vi "meas_gui.vi"() -> ()   [LabVIEW 2015]
doc: "Copyright (c) 2018 Frans Korhonen, Institute for Atmospheric and Earth System Research / Physics, Faculty of Science, University of Helsinki, Finland\n\nThis file is part of MeasGUI.\n\nThis Source Code Form is subject to the terms of the Mozilla Public\nLicense, v. 2.0. If a copy of the MPL was not distributed with this\n file, You can obtain one at http://mozilla.org/MPL/2.0/."
uses:
  <vilib>/Math Plots/3D Math Plots/3D Surface/3D Surface XCtrl/3D Surface.xctl
  <vilib>/Platform/TimedLoop/XDataNode/timing_clust.ctl
  <vilib>/Platform/TimedLoop/XDataNode/nitl_modes.ctl
  <vilib>/Platform/TimedLoop/XDataNode/wakeup.ctl
  <vilib>/Math Plots/3D Math Plots/3D Surface/3D Surface Datatype/Public/Plot Helper (Vector).vi
  <vilib>/platform/TimedLoop/XDataNode/XDataNode.xnode
  <vilib>/Math Plots/3D Math Plots/3D Surface/3D Surface Datatype/3D Surface Datatype.lvclass
  <vilib>/Platform/TimedLoop/XDataNode/XDNodeRunTimeDep.lvlib
  draw_to_matlab.vi
panel:
  out "logged controls":refnum<vi>[](array[refnum])
  out "scan start":u32
  out "program path":path
  out "plot channels":string[](array[string])
  out "graph history":T1(array[cluster])
  out "latest graph data":T1(array[cluster])
  out "saved controls":string[](array[string])=["measurement channels", "measurement comments", "measurement parameters", "measurement settings", "measurement logging", "connection settings", "X channel", "Y channels", "Log x", "Log y", "save measurement", "measurement start commands", "measurement end commands"]
  in  "Tab Control":T2(tab)
  in  "open program folder":bool
  in  "file cluster":T3={"Load"=FALSE, "Save"=FALSE, "Configuration"="test"}
  out "set values":string[][](array[string])
  out "latest":string[](array[string])
  in  "run parameters":T4={"save measurement"=TRUE, "stop count"=0}
  out "graph":T1(graph)=[{"measurement data"=[1.0, 2.333333333333333, 3.6666666666666665, 5.0], "measurement data"=[0.0, 0.0, 0.0, 0.0]}]
  out "start time":timestamp=timestamp(3520583178.0378933 s since 1904-01-01) format="%<%H:%M:%S %p %d.%m.%Y>T"
  in  "Measure":bool
  in  "pause":bool
  in  "stop":bool
  in  "scan":T5(array[cluster])=[{"end"=5.0, "start/single"=1.0, "steps"=5, "list"=[], "measurement type"=1, "set channel"="x"}] {"measurement type" items=["Single", "Linear ramp", "Logarithmic ramp", "Chosen list"]; "list" format="%#_6p"; "start/single" format="%#_6p"; "end" format="%#_6p"}
  out "total steps":i32
  in  "plot to Matlab":bool
  in  "scatter to Matlab":bool
  in  "measurement parameters":T6={"startup wait"=0.0, "settling time"=1.0, "total meas time"=10.0, "meas time"=0.0, "dimensons"=1}
  in  "graph parameters":T7={"X channel"=1, "Y channels"=[2], "Log y"=FALSE, "graph history"=0, "Log x"=FALSE, "auto update"=FALSE} {"Y channels" items=["elapsed", "x", "ad1", "r"]; "X channel" items=["elapsed", "x", "ad1", "r"]}
  out "late from schedule":dbl
  in  "record channels":string[](array[string])
  in  "measurement comments":string="these are the comments for the measurement\nsecond line"
  in  "measurement start commands":string
  in  "measurement end commands":string
  in  "measurement logging":T8={"measurement file"="data\\meas_%Y%m%d", "column separator"=";"}
  in  "next configuration":T9={"load next"=FALSE, "next configuration"="test"}
  out "data":string
  in  "Configure measurement devices":bool
  in  "Configure local hardware":bool
  in  "connection settings":T10={"Serial port"="COM1", "Network address"="192.168.10.15", "connection method"=enum."SERIAL (VISA)", "Port"=1300, "Pipe name"="\\\\.\\pipe\\channel_system"}
  in  "3D graph parameters":T11={"3D X channel"=1, "3D Y channel"=2, "3D Z channel"=3, "auto update"=FALSE} {"3D Z channel" items=["elapsed", "x", "ad1", "r"]; "3D Y channel" items=["elapsed", "x", "ad1", "r"]; "3D X channel" items=["elapsed", "x", "ad1", "r"]}
  out "3D Surface":refnum<class "3D Plot Datatype.lvclass">[](xcontrol)
  in  "draw to matlab":bool
  out "measurement data":dbl[][](array[numeric]) format="%#_3p"
  out "measurement channels":string[](array[string])
  # "click on graph to update manually"
  # "time indicators in filename:\n%Y = year\n%m = month\n%d = day\n%H = hour\n%M = minute\n%S = second"
  # "ms"
  # "0 = dont stop"
  # "+(.csv & .log)"
  # "click on graph to update"
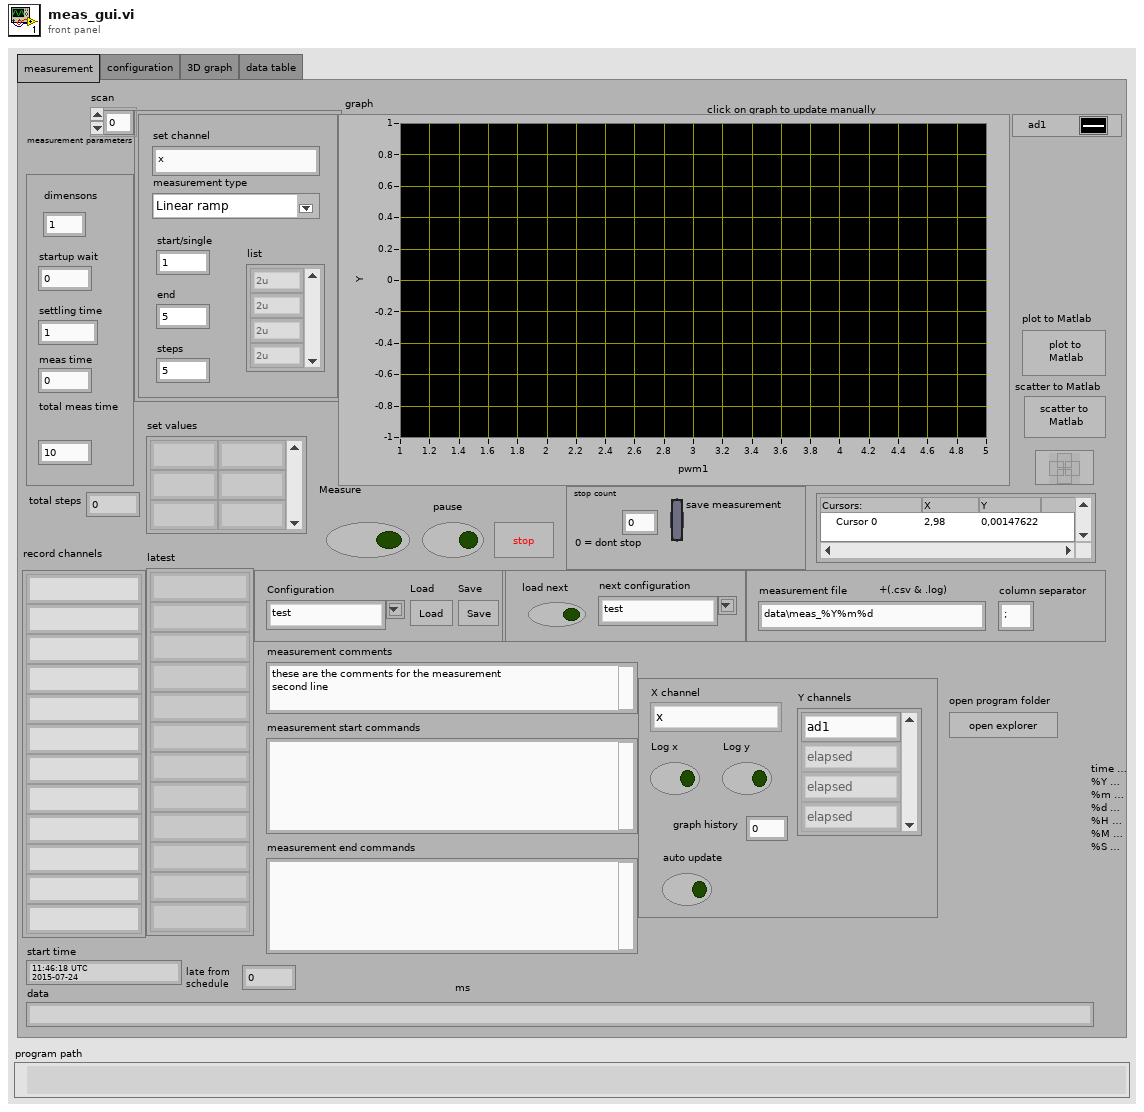
[diagram p1: front panel]
types:
  T1 = cluster{"measurement data":dbl[], "measurement data":dbl[]}[]
  T2 = enum32{"measurement", "configuration", "3D graph", "data table"}
  T3 = cluster{"Load":bool, "Save":bool, "Configuration":string}
  T4 = cluster{"save measurement":bool, "stop count":u32}
  T5 = cluster{"end":dbl, "start/single":dbl, "steps":i32, "list":dbl[], "measurement type":u16, "set channel":string}[]
  T6 = cluster{"startup wait":dbl, "settling time":dbl, "total meas time":dbl, "meas time":dbl, "dimensons":i32}
  T7 = cluster{"X channel":u16, "Y channels":u16[], "Log y":bool, "graph history":i32, "Log x":bool, "auto update":bool}
  T8 = cluster{"measurement file":string, "column separator":string}
  T9 = cluster{"load next":bool, "next configuration":string}
  T10 = cluster{"Serial port":refnum<visa-resource-name>, "Network address":string, "connection method":enum16{"SERIAL (VISA)", "UDP", "LOCAL", "PIPE", "SERIAL (pipe channel)"}, "Port":u16, "Pipe name":string}
  T11 = cluster{"3D X channel":u16, "3D Y channel":u16, "3D Z channel":u16, "auto update":bool}
  T12 = enum16{"open", "replace", "create", "open or create", "replace or create", "replace or create with confirmation"}
  T13 = enum16{"SERIAL (VISA)", "UDP", "LOCAL", "PIPE", "SERIAL (pipe channel)"}
  T14 = cluster{"measurement data":dbl[], "measurement data":dbl[]}
  T15 = enum16{"read", "write", "reset", "conf", "link", "raw communication"}
  T16 = typedef "XDNodeRunTimeDep.lvlib/timing_clust.ctl" = cluster{"Expected End [f-1]":u64, "Actual End [f-1]":u64, "Finished Late? [f-1]":bool, "Expected End [i-1]":u64, "Actual End [i-1]":u64, "Finished Late? [i-1]":bool, "Expected Start [i]":u64, "Actual Start [i]":u64, "Expected Start [f]":u64, "Actual Start [f]":u64, "Source Name":string, "Structure Name":string, "Period":i64, "Deadline":i64, "Offset":i64, "Start":i64, "Priority":i32, "Timeout":i32, "Mode":T17, "Wakeup Reason":T18, "Error":errorcluster, "Source Type":string, "Secondary Source Type":string, "Global End Time":u64, "Global Start Time":u64, "Frame Duration":u64, "Iteration Duration":u64, "Assigned CPU":i32, "I/O Scan Engine Mode":u32}
  T17 = typedef "XDNodeRunTimeDep.lvlib/nitl_modes.ctl" = enum32{"No Change", "Process missed periods, maintain original phase", "Discard missed periods, maintain original phase", "Process missed periods, ignore original phase", "Discard missed periods, ignore original phase"}
  T18 = typedef "XDNodeRunTimeDep.lvlib/wakeup.ctl" = enum32{"Normal", "Aborted", "Asynchronous wakeup", "Timing source error", "Timed loop error", "Timeout"}
  T19 = cluster{"end":dbl, "start/single":dbl, "steps":i32, "list":dbl[], "measurement type":u16, "set channel":string}
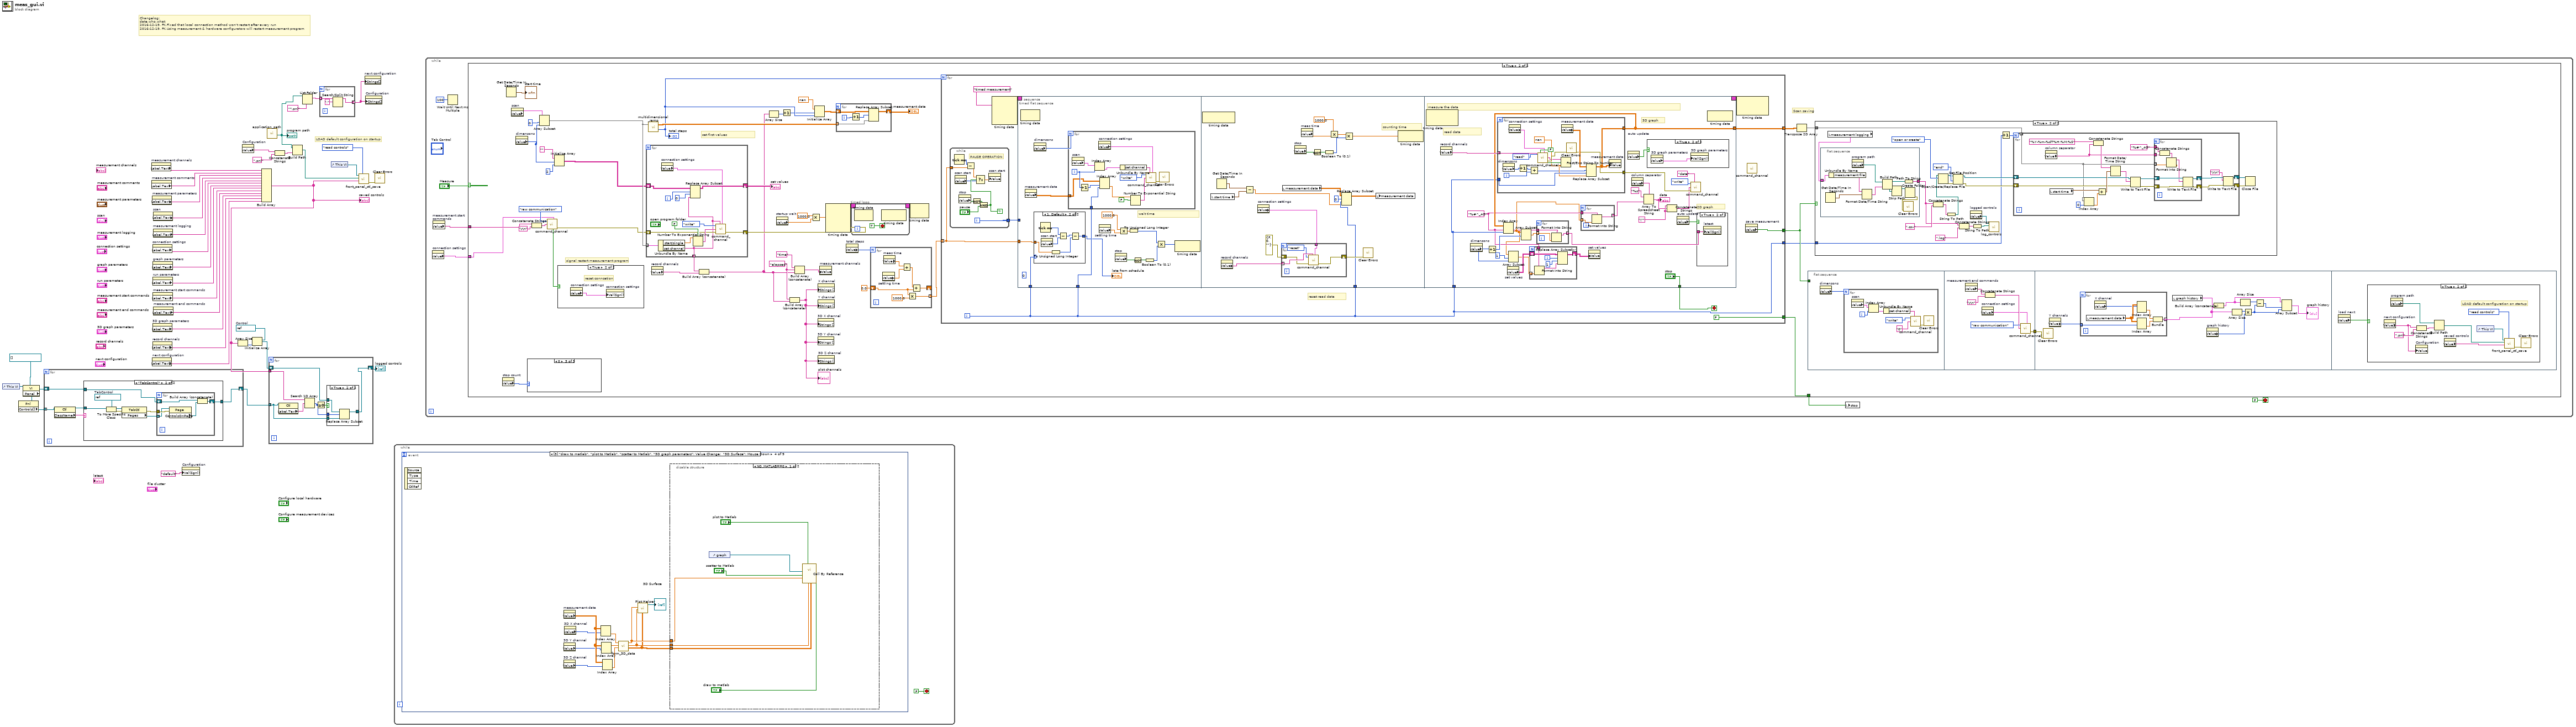
[diagram p0: block diagram]
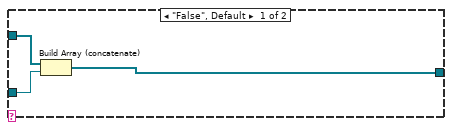
[diagram p3: hidden frame]
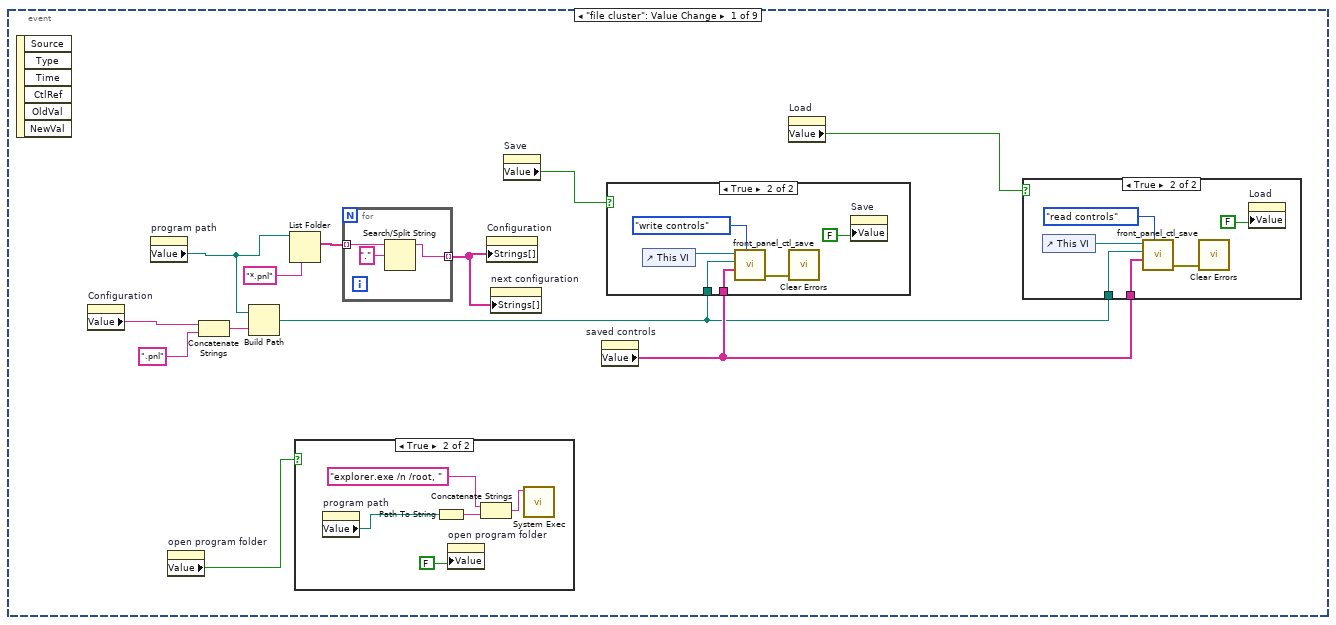
[diagram p4: hidden frame]
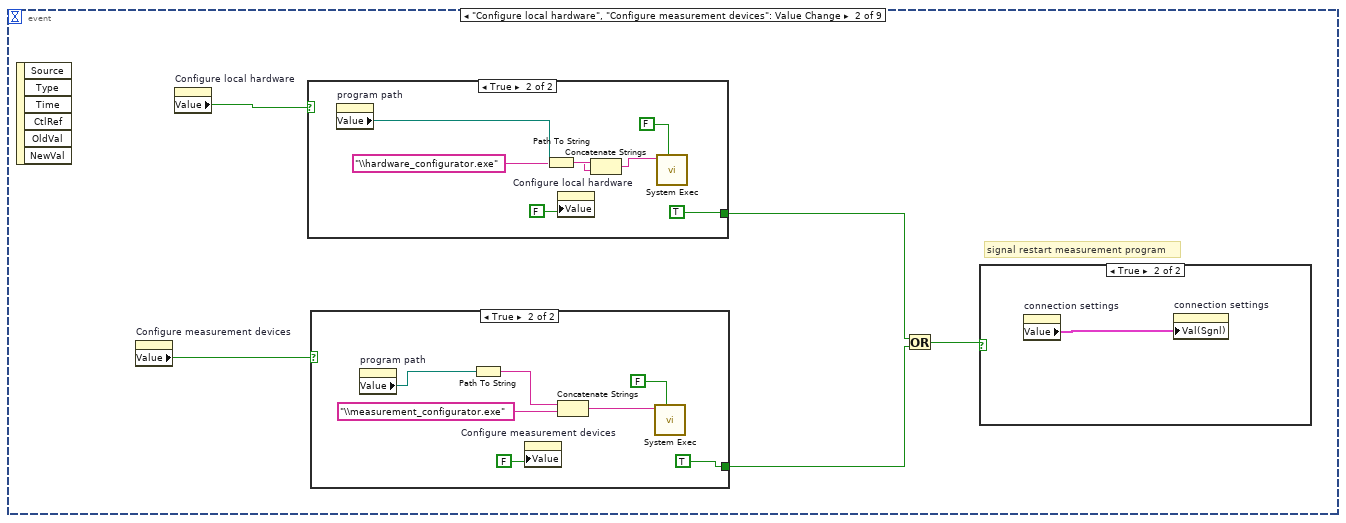
[diagram p8: hidden frame]
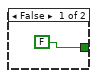
[diagram p10: hidden frame]
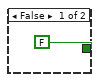
[diagram p11: hidden frame]
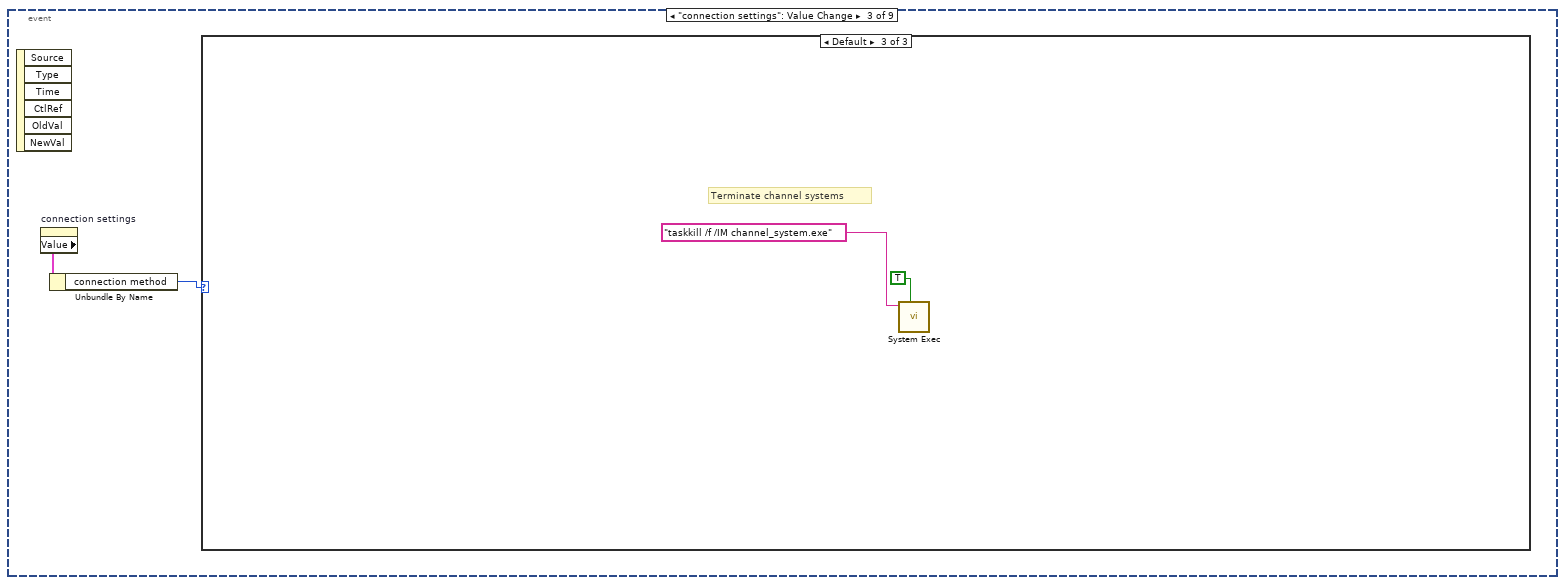
[diagram p12: hidden frame]
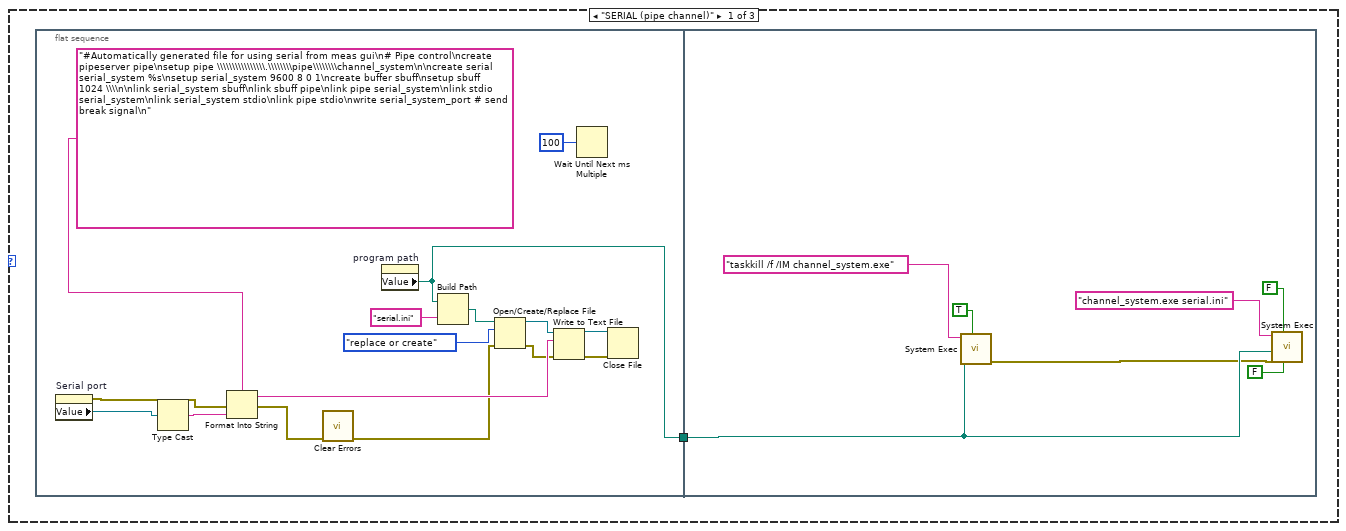
[diagram p13: hidden frame]
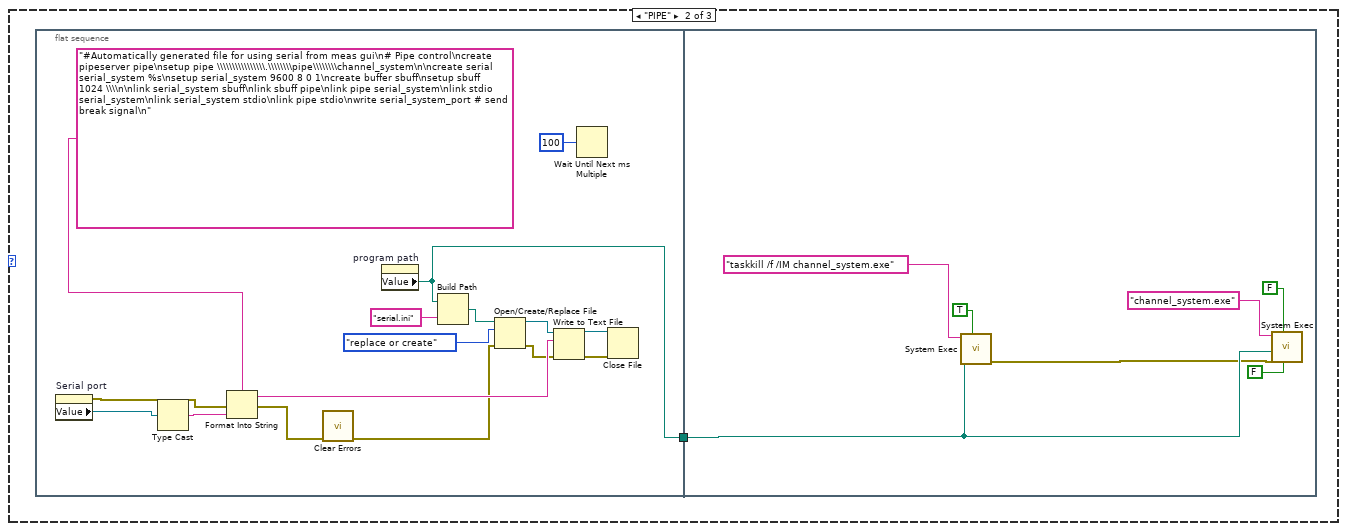
[diagram p14: hidden frame]
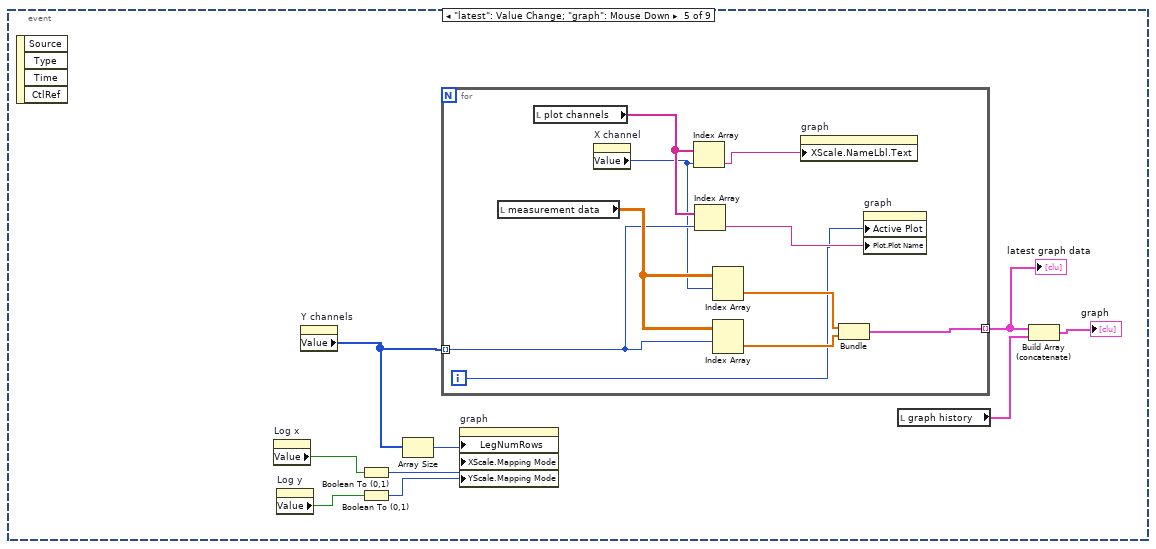
[diagram p16: hidden frame]
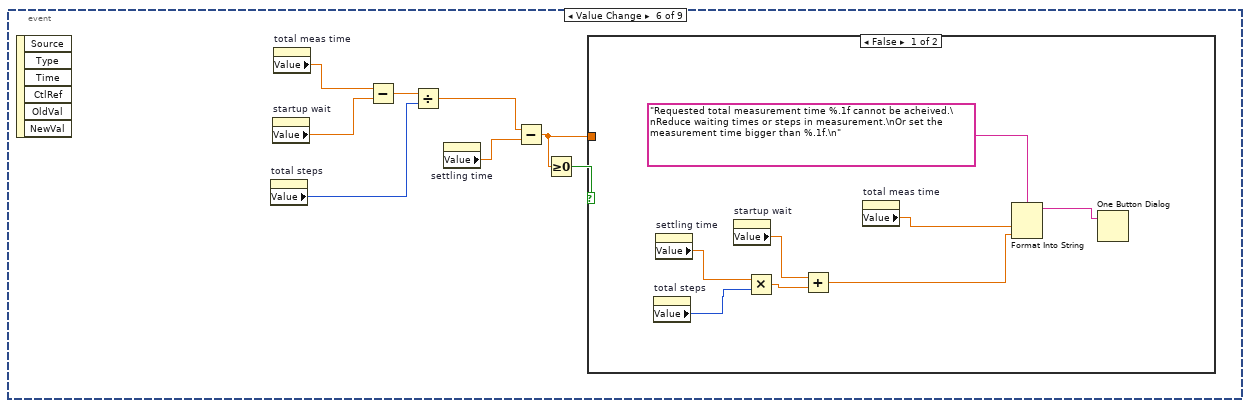
[diagram p17: hidden frame]
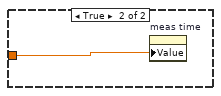
[diagram p18: hidden frame]
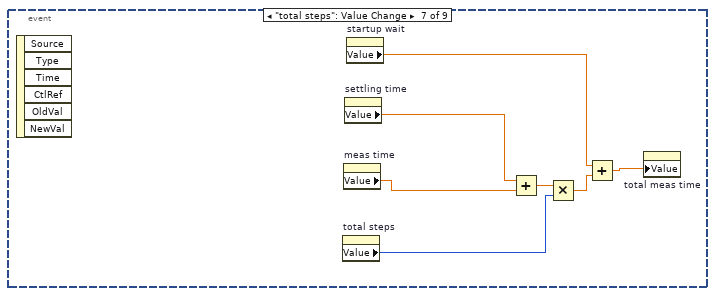
[diagram p19: hidden frame]
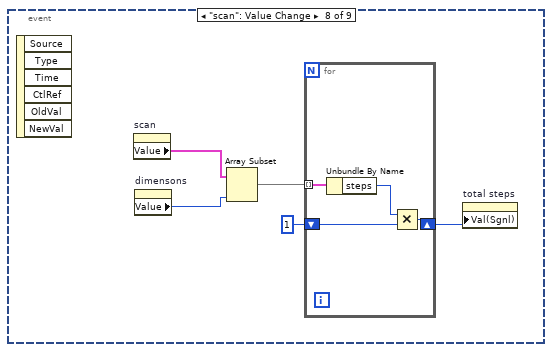
[diagram p20: hidden frame]
diagram:
  w10 = refnum<vi> refnum  # Control
  # "Changelog: \ndate,who,what\n2016-12-19. FK,Fixed that local connection method won't restart after every run\n2016-12-19. FK,Using measurement & hardware configurators will restart measurement program"
  # "LOAD default configuration on startup"
  n1 = control-ref of="This VI"() -> (w17:refnum<vi>)
  n2 = property on="Property Node" class="VI"(reference=w17) -> ("Panel"=w16:refnum<vi>)  [unwired: 1 in, 2 out]
  n3 = property class="Pnl"(reference=w16) -> ("Controls[]"=w15:refnum<vi>[])  [unwired: 1 in, 2 out]
  n4 = for {
    tunnel: w15 -> [w40] mode=indexing
    shift-right: [w37] -> w13
    shift-left: refnum<vi>[] [] -> [w36]
    n5 = property class="Ctl"(reference=w40) -> (reference out=w38:refnum<vi>, "ClassName"=w39:string)  [unwired: 1 in, 1 out]
    n6 = case shown="\"TabControl\"" w39 {
      tunnel: w38 -> [w42 w51]
      tunnel: [w41 w45] -> w37
      tunnel: w36 -> [w43 w44]
      frame "False", Default {
        n7 = Build Array (concatenate)(w43, w42) -> (w41:refnum<vi>[])
      }
      frame "TabControl" {
        w50 = refnum<vi> refnum  # TabControl
        n8 = To More Specific Class(target class=w50, reference=w51) -> (specific class reference=w49:refnum<vi>, error out=w48:errorcluster)  [unwired: 1 in]
        n9 = property class="TabCtl"(reference=w49, error in=w48) -> (error out=w47:errorcluster, "Pages"=w46:refnum<vi>[])  [unwired: 1 out]
        n10 = for {
          tunnel: w47 -> [w56]
          tunnel: w46 -> [w55] mode=indexing
          shift-right: [w53] -> w45
          shift-left: w44 -> [w52]
          n11 = property class="Page"(reference=w55, error in=w56) -> ("ControlsOnPage"=w54:refnum<vi>[])  [unwired: 2 out]
          n12 = Build Array (concatenate)(w52, w54) -> (w53:refnum<vi>[])
        }
      }
    }
  }
  n13 = property on="measurement channels" class="Arr (strict)"() -> ("Label.Text"=w29:string)  [unwired: 2 in, 2 out]
  n14 = property on="measurement comments" class="Str"() -> ("Label.Text"=w27:string)  [unwired: 2 in, 2 out]
  n15 = property on="measurement parameters" class="Clust (strict)"() -> ("Label.Text"=w26:string)  [unwired: 2 in, 2 out]
  n16 = property on="next configuration" class="Clust (strict)"() -> ("Label.Text"=w2:string)  [unwired: 2 in, 2 out]
  n17 = property on="connection settings" class="Clust (strict)"() -> ("Label.Text"=w3:string)  [unwired: 2 in, 2 out]
  n18 = property on="3D graph parameters" class="Clust (strict)"() -> ("Label.Text"=w19:string)  [unwired: 2 in, 2 out]
  n19 = property on="record channels" class="Arr (strict)"() -> ("Label.Text"=w18:string)  [unwired: 2 in, 2 out]
  n20 = property on="graph parameters" class="Clust (strict)"() -> ("Label.Text"=w23:string)  [unwired: 2 in, 2 out]
  n21 = property on="run parameters" class="Clust (strict)"() -> ("Label.Text"=w22:string)  [unwired: 2 in, 2 out]
  n22 = property on="measurement start commands" class="Str"() -> ("Label.Text"=w21:string)  [unwired: 2 in, 2 out]
  n23 = property on="scan" class="Arr (strict)"() -> ("Label.Text"=w25:string)  [unwired: 2 in, 2 out]
  n24 = property on="measurement logging" class="Clust (strict)"() -> ("Label.Text"=w24:string)  [unwired: 2 in, 2 out]
  n25 = property on="measurement end commands" class="Str"() -> ("Label.Text"=w20:string)  [unwired: 2 in, 2 out]
  n26 = property on="Configuration" class="CmbBox"("Val(Sgnl)"="default" ("Value (Signaling)")) -> ()  [unwired: 2 in, 2 out]
  n27 = property on="Configuration" class="CmbBox"() -> ("Value"=w28:string)  [unwired: 2 in, 2 out]
  n28 = Build Array(w29, w27, w26, w25, w24, w3, w23, w22, w21, w20, w19, w18, w2) -> (w12:string[])
  "saved controls" <- w12
  n29 = Array Size(array=w12) -> (size(s)=w11:i32)
  n30 = Initialize Array(w10, w11) -> (w9:refnum<vi>[])
  n31 = call "application_path.vi"() -> ("path"=w4:path)  [unwired: 11 in]
  "program path" <- w4
  n32 = for {
    tunnel: w13 -> [w59] mode=indexing
    tunnel: w12 -> [w62]
    shift-right: [w58] -> w8
    shift-left: w9 -> [w57]
    n33 = property class="Ctl"(reference=w59) -> ("Label.Text"=w63:string)  [unwired: 1 in, 2 out]
    n34 = Search 1D Array(1D array=w62, element=w63) -> (index of element=w60:i32)  [unwired: 1 in]
    n35 = Greater Or Equal To 0?(x=w60) -> (x >= 0?=w61:bool)
    n36 = case shown="True" w61 {
      tunnel: w60 -> [_ w68]
      tunnel: w59 -> [_ w67]
      tunnel: [w64 w66] -> w58
      tunnel: w57 -> [w64 w65]
      frame False {
      }
      frame True {
        n37 = Replace Array Subset(array=w65, new element=w67, index=w68) -> (w66:refnum<vi>[])
      }
    }
  }
  "logged controls" <- w8
  n38 = Concatenate Strings(w28, ".pnl" ("string")) -> (w34:string)
  n39 = Build Path(base path=w4, name or relative path=w34) -> (appended path=w31:path)
  n40 = List Folder(path=w4, pattern="*.pnl") -> (filenames=w5:string[])  [unwired: 2 in, 3 out]
  n41 = for {
    tunnel: w5 -> [w71] mode=indexing
    tunnel: [w70] -> w1 mode=indexing
    n42 = Search/Split String(string=w71, search string/char (-)=".") -> (substring before match=w70:string)  [unwired: 1 in, 2 out]
  }
  n43 = control-ref of="This VI"() -> (w30:refnum<vi>)
  n44 = call "front_panel_ctl_save.vi"("VI in"=w30, "method"=enum16{"read controls", "write controls"}."read controls", "filename"=w31, "controls"=w12) -> ("error out"=w33:errorcluster)  [unwired: 4 in]
  n45 = property on="next configuration" class="CmbBox"("Strings[]"=w1) -> ()  [unwired: 2 in, 2 out]
  n46 = property on="Configuration" class="CmbBox"("Strings[]"=w1) -> ()  [unwired: 2 in, 2 out]
  n47 = call <vilib>:"Clear Errors.vi"("error in (no error)"=w33) -> ()  [unwired: 5 in, 2 out]
  n48 = while {
    stop <- FALSE stop-if-true
    n49 = event shown="[3] \"draw to matlab\", \"plot to Matlab\", \"scatter to Matlab\", \"3D graph parameters\": Value Change;  \"3D Surface\": Mouse Down" {
      selector: _ -> [_ _ _ _ _ _ _ _ _]
      dyn-events: _ -> [_ _ _ _ _ _ _ _ _]
      timeout: _ -> [_ _ _ _ _ _ _ _ _]
      event "file cluster": Value Change {
        n50 = event-data() -> ()  [unwired: 1 in, 6 out]
        n51 = property on="Configuration" class="CmbBox"() -> ("Value"=w77:string)  [unwired: 2 in, 2 out]
        n52 = property on="program path" class="Path"() -> ("Value"=w78:path)  [unwired: 2 in, 2 out]
        n53 = property on="open program folder" class="Bool (strict)"() -> ("Value"=w74:bool)  [unwired: 2 in, 2 out]
        n54 = Concatenate Strings(w77, ".pnl" ("string")) -> (w82:string)
        n55 = Build Path(base path=w78, name or relative path=w82) -> (appended path=w79:path)
        n56 = List Folder(path=w78, pattern="*.pnl") -> (filenames=w81:string[])  [unwired: 2 in, 3 out]
        n57 = case shown="True" w74 {
          frame False {
          }
          frame True {
            n58 = property on="program path" class="Path"() -> ("Value"=w86:path)  [unwired: 2 in, 2 out]
            n59 = Path To String(path=w86) -> (string=w87:string)
            n60 = property on="open program folder" class="Bool (strict)"("Value"=FALSE) -> ()  [unwired: 2 in, 2 out]
            n61 = Concatenate Strings("explorer.exe /n /root, " ("string"), w87) -> (w88:string)
            n62 = call <vilib>:"System Exec.vi"("command line"=w88) -> ()  [unwired: 7 in, 4 out]
          }
        }
        n63 = for {
          tunnel: w81 -> [w92] mode=indexing
          tunnel: [w91] -> w73 mode=indexing
          n64 = Search/Split String(string=w92, search string/char (-)=".") -> (substring before match=w91:string)  [unwired: 1 in, 2 out]
        }
        n65 = property on="Configuration" class="CmbBox"("Strings[]"=w73) -> ()  [unwired: 2 in, 2 out]
        n66 = property on="next configuration" class="CmbBox"("Strings[]"=w73) -> ()  [unwired: 2 in, 2 out]
        n67 = property on="Save" class="Bool (strict)"() -> ("Value"=w75:bool)  [unwired: 2 in, 2 out]
        n68 = property on="saved controls" class="Arr (strict)"() -> ("Value"=w80:string[])  [unwired: 2 in, 2 out]
        n69 = case shown="True" w75 {
          tunnel: w80 -> [_ w102]
          tunnel: w79 -> [_ w101]
          frame False {
          }
          frame True {
            n70 = control-ref of="This VI"() -> (w104:refnum<vi>)
            n71 = call "front_panel_ctl_save.vi"("VI in"=w104, "method"=enum16{"read controls", "write controls"}."write controls", "filename"=w101, "controls"=w102) -> ("error out"=w99:errorcluster)  [unwired: 4 in]
            n72 = call <vilib>:"Clear Errors.vi"("error in (no error)"=w99) -> ()  [unwired: 5 in, 2 out]
            n73 = property on="Save" class="Bool (strict)"("Value"=FALSE) -> ()  [unwired: 2 in, 2 out]
          }
        }
        n74 = property on="Load" class="Bool (strict)"() -> ("Value"=w76:bool)  [unwired: 2 in, 2 out]
        n75 = case shown="True" w76 {
          tunnel: w80 -> [_ w95]
          tunnel: w79 -> [_ w96]
          frame False {
          }
          frame True {
            n76 = control-ref of="This VI"() -> (w97:refnum<vi>)
            n77 = call "front_panel_ctl_save.vi"("VI in"=w97, "method"=enum16{"read controls", "write controls"}."read controls", "filename"=w96, "controls"=w95) -> ("error out"=w93:errorcluster)  [unwired: 4 in]
            n78 = call <vilib>:"Clear Errors.vi"("error in (no error)"=w93) -> ()  [unwired: 5 in, 2 out]
            n79 = property on="Load" class="Bool (strict)"("Value"=FALSE) -> ()  [unwired: 2 in, 2 out]
          }
        }
      }
      event "Configure local hardware", "Configure measurement devices": Value Change {
        # "signal restart measurement program"
        n80 = event-data() -> ()  [unwired: 1 in, 6 out]
        n81 = property on="Configure measurement devices" class="Bool (strict)"() -> ("Value"=w108:bool)  [unwired: 2 in, 2 out]
        n82 = property on="Configure local hardware" class="Bool (strict)"() -> ("Value"=w109:bool)  [unwired: 2 in, 2 out]
        n83 = case shown="True" w109 {
          tunnel: [FALSE TRUE] -> w106
          frame False {
          }
          frame True {
            n84 = property on="program path" class="Path"() -> ("Value"=w124:path)  [unwired: 2 in, 2 out]
            n85 = Path To String(path=w124) -> (string=w125:string)
            n86 = property on="Configure local hardware" class="Bool (strict)"("Value"=FALSE) -> ()  [unwired: 2 in, 2 out]
            n87 = Concatenate Strings(w125, "\\hardware_configurator.exe" ("string")) -> (w126:string)
            n88 = call <vilib>:"System Exec.vi"("wait until completion? (T)"=FALSE, "command line"=w126) -> ()  [unwired: 6 in, 4 out]
          }
        }
        n89 = case shown="True" w108 {
          tunnel: [FALSE TRUE] -> w105
          frame False {
          }
          frame True {
            n90 = property on="program path" class="Path"() -> ("Value"=w115:path)  [unwired: 2 in, 2 out]
            n91 = Path To String(path=w115) -> (string=w114:string)
            n92 = property on="Configure measurement devices" class="Bool (strict)"("Value"=FALSE) -> ()  [unwired: 2 in, 2 out]
            n93 = Concatenate Strings(w114, "\\measurement_configurator.exe" ("string")) -> (w118:string)
            n94 = call <vilib>:"System Exec.vi"("wait until completion? (T)"=FALSE, "command line"=w118) -> ()  [unwired: 6 in, 4 out]
          }
        }
        n95 = Or(x=w106, y=w105) -> (x .or. y?=w107:bool)
        n96 = case shown="True" w107 {
          frame False {
          }
          frame True {
            n97 = property on="connection settings" class="Clust (strict)"() -> ("Value"=w110:T10)  [unwired: 2 in, 2 out]
            n98 = property on="connection settings" class="Clust (strict)"("Val(Sgnl)"=w110) -> ()  [unwired: 2 in, 2 out]
          }
        }
      }
      event "connection settings": Value Change {
        n99 = event-data() -> ()  [unwired: 1 in, 6 out]
        n100 = property on="connection settings" class="Clust (strict)"() -> ("Value"=w128:T10)  [unwired: 2 in, 2 out]
        n101 = Unbundle By Name(w128) -> ("connection method"=w127:T13)
        n102 = case shown="Default" w127 {
          frame "SERIAL (pipe channel)" {
            n103 = flat-sequence {
              tunnel: [w131] -> w129
              tunnel: w129 -> [w147]
              frame #0 {
                n104 = property on="Serial port" class="VISAName"() -> (error out=w138:errorcluster, "Value"=w136:refnum<visa-resource-name>)  [unwired: 2 in, 1 out]
                n105 = Type Cast(x=w136) -> (*(type *) &x=w137:string)  [unwired: 1 in]
                n106 = Format Into String(format string="#Automatically generated file for using serial from meas gui\n# Pipe control\ncreate pipeserver pipe\nsetup pipe \\\\\\\\\\\\\\\\.\\\\\\\\pipe\\\\\\\\channel_system\n\ncreate serial serial_system %s\nsetup serial_system 9600 8 0 1\ncreate buffer sbuff\nsetup sbuff 1024 \\\\n\nlink serial_system sbuff\nlink sbuff pipe\nlink pipe serial_system\nlink stdio serial_system\nlink serial_system stdio\nlink pipe stdio\nwrite serial_system_port # send break signal\n", error in=w138, w137) -> (resulting string=w144:string, error out=w139:errorcluster)  [unwired: 1 in]
                n107 = call <vilib>:"Clear Errors.vi"("error in (no error)"=w139) -> ("error out"=w133:errorcluster)  [unwired: 5 in, 1 out]
                n108 = property on="program path" class="Path"() -> ("Value"=w131:path)  [unwired: 2 in, 2 out]
                n109 = Build Path(base path=w131, name or relative path="serial.ini") -> (appended path=w141:path)
                n110 = Open/Create/Replace File(file path (use dialog)=w141, error in=w133, operation (0:open)=T12."replace or create") -> (refnum out=w143:refnum<file>, error out=w134:errorcluster)  [unwired: 3 in, 1 out]
                n111 = Write to Text File(file (use dialog)=w143, text=w144, error in=w134) -> (refnum out=w145:refnum<file>, error out=w135:errorcluster)  [unwired: 1 in, 1 out]
                n112 = Wait Until Next ms Multiple(millisecond multiple=u32 100) -> ()  [unwired: 1 out]
                n113 = Close File(refnum=w145, error in=w135) -> ()  [unwired: 2 out]
              }
              frame #1 {
                n114 = call <vilib>:"System Exec.vi"("wait until completion? (T)"=TRUE, "working directory"=w147, "command line"="taskkill /f /IM channel_system.exe") -> ("error out"=w146:errorcluster)  [unwired: 5 in, 3 out]
                n115 = call <vilib>:"System Exec.vi"("run minimized? (F)"=FALSE, "wait until completion? (T)"=FALSE, "error in (no error)"=w146, "working directory"=w147, "command line"="channel_system.exe serial.ini") -> ()  [unwired: 3 in, 4 out]
              }
            }
          }
          frame "PIPE" {
            n116 = flat-sequence {
              tunnel: [w155] -> w153
              tunnel: w153 -> [w171]
              frame #0 {
                n117 = property on="Serial port" class="VISAName"() -> (error out=w162:errorcluster, "Value"=w160:refnum<visa-resource-name>)  [unwired: 2 in, 1 out]
                n118 = Type Cast(x=w160) -> (*(type *) &x=w161:string)  [unwired: 1 in]
                n119 = Format Into String(format string="#Automatically generated file for using serial from meas gui\n# Pipe control\ncreate pipeserver pipe\nsetup pipe \\\\\\\\\\\\\\\\.\\\\\\\\pipe\\\\\\\\channel_system\n\ncreate serial serial_system %s\nsetup serial_system 9600 8 0 1\ncreate buffer sbuff\nsetup sbuff 1024 \\\\n\nlink serial_system sbuff\nlink sbuff pipe\nlink pipe serial_system\nlink stdio serial_system\nlink serial_system stdio\nlink pipe stdio\nwrite serial_system_port # send break signal\n", error in=w162, w161) -> (resulting string=w168:string, error out=w163:errorcluster)  [unwired: 1 in]
                n120 = call <vilib>:"Clear Errors.vi"("error in (no error)"=w163) -> ("error out"=w157:errorcluster)  [unwired: 5 in, 1 out]
                n121 = property on="program path" class="Path"() -> ("Value"=w155:path)  [unwired: 2 in, 2 out]
                n122 = Build Path(base path=w155, name or relative path="serial.ini") -> (appended path=w165:path)
                n123 = Open/Create/Replace File(file path (use dialog)=w165, error in=w157, operation (0:open)=T12."replace or create") -> (refnum out=w167:refnum<file>, error out=w158:errorcluster)  [unwired: 3 in, 1 out]
                n124 = Write to Text File(file (use dialog)=w167, text=w168, error in=w158) -> (refnum out=w169:refnum<file>, error out=w159:errorcluster)  [unwired: 1 in, 1 out]
                n125 = Wait Until Next ms Multiple(millisecond multiple=u32 100) -> ()  [unwired: 1 out]
                n126 = Close File(refnum=w169, error in=w159) -> ()  [unwired: 2 out]
              }
              frame #1 {
                n127 = call <vilib>:"System Exec.vi"("wait until completion? (T)"=TRUE, "working directory"=w171, "command line"="taskkill /f /IM channel_system.exe") -> ("error out"=w170:errorcluster)  [unwired: 5 in, 3 out]
                n128 = call <vilib>:"System Exec.vi"("run minimized? (F)"=FALSE, "wait until completion? (T)"=FALSE, "error in (no error)"=w170, "working directory"=w171, "command line"="channel_system.exe") -> ()  [unwired: 3 in, 4 out]
              }
            }
          }
          frame Default {
            # "Terminate channel systems"
            n129 = call <vilib>:"System Exec.vi"("wait until completion? (T)"=TRUE, "command line"="taskkill /f /IM channel_system.exe") -> ()  [unwired: 6 in, 4 out]
          }
        }
      }
      event "draw to matlab", "plot to Matlab", "scatter to Matlab", "3D graph parameters": Value Change; "3D Surface": Mouse Down {
        n130 = event-data() -> ()  [unwired: 1 in, 4 out]
        n131 = property on="measurement data" class="Arr (strict)"() -> ("Value"=w189:dbl[][])  [unwired: 2 in, 2 out]
        n132 = property on="3D Y channel" class="Ring (strict)"() -> ("Value"=w188:u16)  [unwired: 2 in, 2 out]
        n133 = property on="3D Z channel" class="Ring (strict)"() -> ("Value"=w187:u16)  [unwired: 2 in, 2 out]
        n134 = property on="3D X channel" class="Ring (strict)"() -> ("Value"=w186:u16)  [unwired: 2 in, 2 out]
        n135 = Index Array(array=w189, index (row)=w186) -> (element=w183:dbl[])  [unwired: 1 in]
        n136 = Index Array(array=w189, index (row)=w188) -> (element=w184:dbl[])  [unwired: 1 in]
        n137 = Index Array(array=w189, index (row)=w187) -> (element=w185:dbl[])  [unwired: 1 in]
        n138 = call "form_3D_data.vi"("z data"=w185, "y data"=w184, "x data"=w183) -> ("Z matrix"=w179:dbl[][], "y vector"=w180:dbl[], "x vector"=w181:dbl[])  [unwired: 6 in]
        n139 = call-poly <vilib>:"Plot Helper.vi"("z matrix"=w179, "y vector"=w180, "x vector"=w181) -> ("3D Plot lvclass Array out"=→"3D Surface":refnum<class "3D Plot Datatype.lvclass">[])  [unwired: 3 in, 5 out]
        n140 = disable-structure shown="NO_MATLAB==0" {
          disable-tunnel: w181 -> [w193 _]
          disable-tunnel: w180 -> [w192 _]
          disable-tunnel: w179 -> [w191 _]
          frame condition #0 (active) {
            n141 = control-ref of="graph"() -> (w190:refnum<vi>)
            n142 = call-by-ref "?"("Z matrix"=w191, "draw to matlab"="draw to matlab", "y vector"=w192, "plot to Matlab"="plot to Matlab", "x vector"=w193, "scatter to Matlab"="scatter to Matlab", "XYGraph in"=w190) -> ()  [unwired: 7 in, 2 out]
          }
          frame condition #1 {
          }
        }
      }
      event "latest": Value Change; "graph": Mouse Down {
        n143 = event-data() -> ()  [unwired: 1 in, 4 out]
        n144 = property on="Log x" class="Bool (strict)"() -> ("Value"=w200:bool)  [unwired: 2 in, 2 out]
        n145 = property on="Log y" class="Bool (strict)"() -> ("Value"=w199:bool)  [unwired: 2 in, 2 out]
        n146 = property on="Y channels" class="Arr (strict)"() -> ("Value"=w198:u16[])  [unwired: 2 in, 2 out]
        n147 = Boolean To (0,1)(Boolean=w200) -> (0, 1=w205:i16)
        n148 = Boolean To (0,1)(Boolean=w199) -> (0, 1=w203:i16)
        n149 = Array Size(array=w198) -> (size(s)=w204:i32)
        n150 = for {
          tunnel: [w215] -> w202 mode=indexing
          tunnel: w198 -> [w210] mode=indexing
          i -> [w207]
          n151 = local read "measurement data"() -> (w214:dbl[][])
          n152 = local read "plot channels"() -> (w211:string[])
          n153 = property on="X channel" class="Ring (strict)"() -> ("Value"=w206:u16)  [unwired: 2 in, 2 out]
          n154 = Index Array(array=w211, index=w206) -> (element=w209:string)
          n155 = Index Array(array=w211, index=w210) -> (element=w208:string)
          n156 = Index Array(array=w214, index (row)=w206) -> (element=w213:dbl[])  [unwired: 1 in]
          n157 = Index Array(array=w214, index (row)=w210) -> (element=w212:dbl[])  [unwired: 1 in]
          n158 = property on="graph" class="XYGraph (strict)"("XScale.NameLbl.Text"=w209) -> ()  [unwired: 2 in, 2 out]
          n159 = Bundle("measurement data"=w213, "measurement data"=w212) -> (w215:T14)  [unwired: 1 in]
          n160 = property on="graph" class="XYGraph (strict)"("Active Plot"=w207, "Plot.Plot Name"=w208) -> ()  [unwired: 2 in, 2 out]
        }
        "latest graph data" <- w202
        n161 = property on="graph" class="XYGraph (strict)"("LegNumRows"=w204, "XScale.Mapping Mode"=w205, "YScale.Mapping Mode"=w203) -> ()  [unwired: 2 in, 2 out]
        n162 = local read "graph history"() -> (w201:T1)
        n163 = Build Array (concatenate)(w202, w201) -> (→"graph":T1)
      }
      event "measurement parameters.total meas time": Value Change {
        n164 = event-data() -> ()  [unwired: 1 in, 6 out]
        n165 = property on="total steps" class="DigNum (strict)"() -> ("Value"=w220:i32)  [unwired: 2 in, 2 out]
        n166 = property on="startup wait" class="DigNum (strict)"() -> ("Value"=w222:dbl)  [unwired: 2 in, 2 out]
        n167 = property on="total meas time" class="DigNum (strict)"() -> ("Value"=w223:dbl)  [unwired: 2 in, 2 out]
        n168 = Subtract(x=w223, y=w222) -> (x-y=w221:dbl)
        n169 = Divide(x=w221, y=w220) -> (x/y=w218:dbl)
        n170 = property on="settling time" class="DigNum (strict)"() -> ("Value"=w219:dbl)  [unwired: 2 in, 2 out]
        n171 = Subtract(x=w218, y=w219) -> (x-y=w216:dbl)
        n172 = Greater Or Equal To 0?(x=w216) -> (x >= 0?=w217:bool)
        n173 = case shown="False" w217 {
          tunnel: w216 -> [_ w232]
          frame False {
            n174 = property on="total steps" class="DigNum (strict)"() -> ("Value"=w228:i32)  [unwired: 2 in, 2 out]
            n175 = property on="settling time" class="DigNum (strict)"() -> ("Value"=w229:dbl)  [unwired: 2 in, 2 out]
            n176 = property on="startup wait" class="DigNum (strict)"() -> ("Value"=w227:dbl)  [unwired: 2 in, 2 out]
            n177 = Multiply(x=w229, y=w228) -> (x*y=w226:dbl)
            n178 = Add(x=w227, y=w226) -> (x+y=w225:dbl)
            n179 = property on="total meas time" class="DigNum (strict)"() -> ("Value"=w230:dbl)  [unwired: 2 in, 2 out]
            n180 = Format Into String(format string="Requested total measurement time %.1f cannot be acheived.\nReduce waiting times or steps in measurement.\nOr set the measurement time bigger than %.1f.\n", w230, w225) -> (resulting string=w224:string)  [unwired: 2 in, 1 out]
            n181 = One Button Dialog(message=w224) -> ()  [unwired: 1 in, 1 out]
          }
          frame True {
            n182 = property on="meas time" class="DigNum (strict)"("Value"=w232) -> ()  [unwired: 2 in, 2 out]
          }
        }
      }
      event "measurement parameters.meas time", "total steps", "measurement parameters.settling time", "measurement parameters.startup wait": Value Change {
        n183 = event-data() -> ()  [unwired: 1 in, 6 out]
        n184 = property on="total steps" class="DigNum (strict)"() -> ("Value"=w234:i32)  [unwired: 2 in, 2 out]
        n185 = property on="meas time" class="DigNum (strict)"() -> ("Value"=w238:dbl)  [unwired: 2 in, 2 out]
        n186 = property on="settling time" class="DigNum (strict)"() -> ("Value"=w239:dbl)  [unwired: 2 in, 2 out]
        n187 = property on="startup wait" class="DigNum (strict)"() -> ("Value"=w237:dbl)  [unwired: 2 in, 2 out]
        n188 = Add(x=w239, y=w238) -> (x+y=w236:dbl)
        n189 = Multiply(x=w236, y=w234) -> (x*y=w235:dbl)
        n190 = Add(x=w237, y=w235) -> (x+y=w233:dbl)
        n191 = property on="total meas time" class="DigNum (strict)"("Value"=w233) -> ()  [unwired: 2 in, 2 out]
      }
      event "scan", "measurement parameters.dimensons": Value Change {
        n192 = event-data() -> ()  [unwired: 1 in, 6 out]
        n193 = property on="scan" class="Arr (strict)"() -> ("Value"=w244:T5)  [unwired: 2 in, 2 out]
        n194 = property on="dimensons" class="DigNum (strict)"() -> ("Value"=w243:i32)  [unwired: 2 in, 2 out]
        n195 = Array Subset(array=w244, length=w243) -> (w242:T5)  [unwired: 1 in]
        n196 = for {
          tunnel: w242 -> [w248] mode=indexing
          shift-right: [w245] -> w240
          shift-left: 1 -> [w246]
          n197 = Unbundle By Name(w248) -> ("steps"=w247:i32)
          n198 = Multiply(x=w247, y=w246) -> (x*y=w245:i32)
        }
        n199 = property on="total steps" class="DigNum (strict)"("Val(Sgnl)"=w240) -> ()  [unwired: 2 in, 2 out]
      }
      event "stop": Value Change {
        n200 = event-data() -> ()  [unwired: 1 in, 6 out]
        n201 = call <vilib>:"Stop Timed Structure.vi"("name"="timed measurement") -> ("error out"=w249:errorcluster)  [unwired: 10 in]
        n202 = call <vilib>:"Clear Errors.vi"("error in (no error)"=w249) -> ()  [unwired: 5 in, 2 out]
      }
    }
  }
  n203 = while {
    stop <- FALSE stop-if-true
    n204 = property on="connection settings" class="Clust (strict)"() -> ("Value"=w251:T10)  [unwired: 2 in, 2 out]
    n205 = property on="measurement start commands" class="Str"() -> ("Value"=w253:string)  [unwired: 2 in, 2 out]
    n206 = Wait Until Next ms Multiple(millisecond multiple=u32 100) -> ()  [unwired: 1 out]
    n207 = case shown="True" "Measure" {
      tunnel: [FALSE ("stop") w297] -> w255
      tunnel: w253 -> [_ w286]
      tunnel: w251 -> [_ w263]
      frame False {
        (unwired) TRUE ("stop 2")
        n208 = property on="Numeric" class="DigNum (strict)"() -> ("NumText.Height"=w257:u32)  [unwired: 2 in, 2 out]
        n209 = property on="String" class="Str"("Height"=w257) -> ()  [unwired: 2 in, 2 out]
      }
      frame True {
        w294 = "elapsed"
        # "signal restart measurement program"
        # "Scan saving"
        # "set first values"
        n210 = property on="stop count" class="DigNum (strict)"() -> ("Value"=w290:u32)  [unwired: 2 in, 2 out]
        n211 = Get Date/Time In Seconds() -> (seconds since 1Jan1904=→"start time":timestamp)
        n212 = property on="scan" class="Arr (strict)"() -> ("Value"=w291:T5)  [unwired: 2 in, 2 out]
        n213 = property on="dimensons" class="DigNum (strict)"() -> ("Value"=w267:i32)  [unwired: 2 in, 2 out]
        n214 = case shown="0" w290 {
          selector: w290 -> [w381 w383 _]
          frame Default {
            n215 = Decrement(x=w381) -> (x-1=w380:u32)
            n216 = property on="stop count" class="DigNum (strict)"("Value"=w380) -> ()  [unwired: 2 in, 2 out]
          }
          frame 1 {
            n217 = Decrement(x=w383) -> (x-1=w384:u32)
            n218 = property on="stop count" class="DigNum (strict)"("Value"=w384) -> ()  [unwired: 2 in, 2 out]
            n219 = property on="Measure" class="Bool (strict)"("Value"=FALSE ("Measure")) -> ()  [unwired: 2 in, 2 out]
          }
          frame 0 {
          }
        }
        n220 = Concatenate Strings(w286, "\r\n") -> (w298:string)
        n221 = Array Subset(array=w291, index=0, length=w267) -> (w287:T5)
        n222 = call "command_channel.vi"("command"=T15."raw communication", "data"=w298, "connection settings"=w263) -> ("no connection"=w261:bool, "error out"=w262:errorcluster)  [unwired: 4 in, 1 out]
        n223 = Initialize Array("", w267, 2 ("dimension size")) -> (w266:string[][])
        n224 = case shown="True" w261 {
          frame False {
          }
          frame True {
            # "reset conncetion"
            n225 = property on="connection settings" class="Clust (strict)"() -> ("Value"=w305:T10)  [unwired: 2 in, 2 out]
            n226 = property on="connection settings" class="Clust (strict)"("Val(Sgnl)"=w305) -> ()  [unwired: 2 in, 2 out]
          }
        }
        n227 = for {
          tunnel: [w328] -> w296 mode=indexing
          tunnel: w287 -> [w333] mode=indexing
          shift-right: [w335] -> w276
          shift-left: w262 -> [w332]
          shift-right: [w327] -> w265
          shift-left: w266 -> [w331]
          i -> [w330]
          n228 = Unbundle By Name(w333) -> ("start/single"=w334:dbl, "set channel"=w328:string)
          n229 = property on="connection settings" class="Clust (strict)"() -> ("Value"=w326:T10)  [unwired: 2 in, 2 out]
          n230 = Replace Array Subset(array=w331, new element=w328, index (row)=w330, index (col)=0 ("disabled index (col)")) -> (w327:string[][])
          n231 = Number To Exponential String(number=w334, 1:FALSE ("use system decimal point (T)")) -> (E-format string=w337:string)  [unwired: 2 in]
          n232 = call "command_channel.vi"("command"=enum16{"read", "write", "reset", "conf", "link"}."write", "channel"=w328, "data"=w337, "error in"=w332, "connection settings"=w326) -> ("error out"=w335:errorcluster)  [unwired: 2 in, 2 out]
        }
        "set values" <- w265
        n233 = call "multidimensional_ramp.vi"("params"=w287) -> ("steps"=w282:i32, "multidimensional ramp"=w283:dbl[][])  [unwired: 1 in]
        "total steps" <- w282
        n234 = property on="record channels" class="Arr (strict)"() -> ("Value"=w288:string[])  [unwired: 2 in, 2 out]
        n235 = Build Array (concatenate)(w296, w288) -> (w264:string[])
        n236 = Array Size(array=w264) -> (size(s)=w301:i32)
        n237 = property on="startup wait" class="DigNum (strict)"() -> ("Value"=w280:dbl)  [unwired: 2 in, 2 out]
        n238 = Increment(x=w301) -> (x+1=w259:i32)
        n239 = Build Array (concatenate)(w294, w264) -> (w293:string[])
        "plot channels" <- w293
        n240 = Build Array (concatenate)("time", w294, w264) -> (w289:string[])
        n241 = Multiply(x=1000.0, y=w280) -> (x*y=w277:dbl)
        n242 = Initialize Array(nan, w259, w282) -> (w284:dbl[][])
        n243 = property on="3D X channel" class="Ring (strict)"("Strings []"=w293) -> ()  [unwired: 2 in, 2 out]
        n244 = property on="3D Y channel" class="Ring (strict)"("Strings []"=w293) -> ()  [unwired: 2 in, 2 out]
        n245 = property on="X channel" class="Ring (strict)"("Strings []"=w293) -> ()  [unwired: 2 in, 2 out]
        n246 = property on="Y channel" class="Ring (strict)"("Strings []"=w293) -> ()  [unwired: 2 in, 2 out]
        n247 = property on="3D Z channel" class="Ring (strict)"("Strings []"=w293) -> ()  [unwired: 2 in, 2 out]
        n248 = property on="measurement channels" class="Arr (strict)"("Value"=w289) -> ()  [unwired: 2 in, 2 out]
        n249 = node-c288(w277, w276) -> (w279:T16)  [unwired: 2 in]
        n250 = for {
          tunnel: w283 -> [w325] mode=indexing
          shift-right: [w323] -> w273
          shift-left: w284 -> [w322]
          i -> [w324]
          n251 = Increment(x=w324) -> (x+1=w321:i32)
          n252 = Replace Array Subset(array=w322, new element=w325, index (row)=w321) -> (w323:dbl[][])  [unwired: 1 in]
        }
        "measurement data" <- w273
        n253 = property on="total steps" class="DigNum (strict)"() -> ("Value"=w271:i32)  [unwired: 2 in, 2 out]
        n254 = timed-loop {
          timing: w279 -> [_]
          timing-out: [_] -> w278
          stop <- TRUE stop-if-true
          n255 = node-c288() -> ()  [unwired: 1 in, 1 out]
          n256 = node-c288() -> ()  [unwired: 1 in, 1 out]
        }
        n257 = for {
          N: w271 -> [_]
          shift-right: [w308] -> _
          shift-left: 0.0 -> [w307]
          tunnel: [w306] -> w270 mode=indexing
          n258 = property on="settling time" class="DigNum (strict)"() -> ("Value"=w310:dbl)  [unwired: 2 in, 2 out]
          n259 = property on="meas time" class="DigNum (strict)"() -> ("Value"=w309:dbl)  [unwired: 2 in, 2 out]
          n260 = Add(x=w309, y=w310) -> (x+y=w311:dbl)
          n261 = Multiply(x=w307, y=1000.0) -> (x*y=w306:dbl)
          n262 = Add(x=w311, y=w307) -> (x+y=w308:dbl)
        }
        n263 = node-c288(w278) -> ()  [unwired: 1 out]
        n264 = for {
          N: w282 -> [_]
          tunnel: [w451] -> w302
          tunnel: [FALSE ("stop")] -> w297
          tunnel: [w449] -> w274
          tunnel: w270 -> [w443] mode=indexing
          tunnel: [w442] -> w260
          i -> [w442]
          stop <- w444 stop-if-true
          # "reset read data"
          n265 = while {
            tunnel: [w461] -> w446
            tunnel: w443 -> [w455]
            i -> [w461]
            stop <- w457 continue-if-true
            # "PAUSE OPERATION"
            n266 = Tick Count (ms)() -> (millisecond timer value=w454:u32)
            n267 = property on="scan start" class="DigNum (strict)"() -> ("Value"=w456:u32)  [unwired: 2 in, 2 out]
            n268 = property on="stop" class="Bool (strict)"() -> ("Value"=w459:bool)  [unwired: 2 in, 2 out]
            n269 = Subtract(x=w454, y=w455) -> (x-y=w453:dbl)
            n270 = Not(x=w459) -> (.not. x?=w460:bool)
            n271 = And(x=w460, y="pause") -> (x .and. y?=w457:bool)
            n272 = Select(t=w453, s=w457, f=w456) -> (s? t:f=w452:dbl)
            n273 = property on="scan start" class="DigNum (strict)"("Value"=w452) -> ()  [unwired: 2 in, 2 out]
          }
          n274 = node-c288("timed measurement" ("Structure Name")) -> (w448:T16)  [unwired: 3 in]
          n275 = timed-sequence {
            timing: w448 -> [_]
            timing-out: [_] -> w447
            tunnel: w442 -> [w469]
            tunnel: [w468] -> w451
            tunnel: w442 -> [w467]
            tunnel: w446 -> [w466]
            tunnel: [w465] -> w444
            tunnel: w442 -> [w464]
            tunnel: w443 -> [w462]
            tunnel: w442 -> [w463]
            n276 = timed-flat-sequence {
              tunnel: w466 -> [_]
              tunnel: w464 -> [w477]
              tunnel: w463 -> [w476]
              tunnel: w462 -> [w472]
              tunnel: w469 -> [w524]
              tunnel: [w548] -> w468
              tunnel: w467 -> [w547]
              tunnel: ["stop"] -> w465
              frame #0 {
                (unwired) u32 0 ("millisecond timer value")
                # "wait time"
                n277 = node-c288() -> ()  [unwired: 1 in, 1 out]
                n278 = property on="measurement data" class="Arr (strict)"() -> ("Value"=w478:dbl[][])  [unwired: 2 in, 2 out]
                n279 = case shown="1, Default" w476 {
                  tunnel: [u32 0 ("millisecond timer value") w489] -> w473
                  tunnel: w472 -> [_ w486]
                  frame 0 {
                    n280 = Tick Count (ms)() -> (millisecond timer value=→"scan start":u32)
                  }
                  frame 1, Default {
                    n281 = Tick Count (ms)() -> (millisecond timer value=w491:u32)
                    n282 = property on="scan start" class="DigNum (strict)"() -> ("Value"=w490:u32)  [unwired: 2 in, 2 out]
                    n283 = To Unsigned Long Integer(number=w486) -> (unsigned 32bit integer=w487:u32)
                    n284 = Subtract(x=w491, y=w490) -> (x-y=w488:u32)
                    n285 = Subtract(x=w488, y=w487) -> (x-y=w489:u32)
                  }
                }
                "late from schedule" <- w473
                n286 = property on="dimensons" class="DigNum (strict)"() -> ("Value"=w479:i32)  [unwired: 2 in, 2 out]
                n287 = for {
                  N: w479 -> [_]
                  tunnel: w478 -> [w500]
                  tunnel: w477 -> [w497]
                  i -> [w501]
                  n288 = property on="scan" class="Arr (strict)"() -> ("Value"=w503:T5)  [unwired: 2 in, 2 out]
                  n289 = Increment(x=w501) -> (x+1=w498:i32)
                  n290 = Index Array(array=w503, index=w501) -> (element=w502:T19)
                  n291 = property on="connection settings" class="Clust (strict)"() -> ("Value"=w496:T10)  [unwired: 2 in, 2 out]
                  n292 = Index Array(array=w500, index (row)=w498, index (col)=w497) -> (element=w499:dbl)
                  n293 = Unbundle By Name(w502) -> ("set channel"=w508:string)
                  n294 = Number To Exponential String(number=w499, 1:FALSE ("use system decimal point (T)")) -> (E-format string=w507:string)  [unwired: 2 in]
                  n295 = call "command_channel.vi"("command"=enum16{"read", "write", "reset", "conf", "link"}."write", "channel"=w508, "data"=w507, "connection settings"=w496) -> ("error out"=w506:errorcluster)  [unwired: 3 in, 2 out]
                  n296 = call <vilib>:"Clear Errors.vi"("error in (no error)"=w506) -> ()  [unwired: 5 in, 2 out]
                }
                n297 = property on="settling time" class="DigNum (strict)"() -> ("Value"=w475:dbl)  [unwired: 2 in, 2 out]
                n298 = property on="stop" class="Bool (strict)"() -> ("Value"=w482:bool)  [unwired: 2 in, 2 out]
                n299 = Multiply(x=1000.0, y=w475) -> (x*y=w471:dbl)
                n300 = To Unsigned Long Integer(number=w471) -> (unsigned 32bit integer=w470:u32)
                n301 = Not(x=w482) -> (.not. x?=w483:bool)
                n302 = Boolean To (0,1)(Boolean=w483) -> (0, 1=w481:i16)
                n303 = Multiply(x=w470, y=w481) -> (x*y=w480:u32)
                n304 = node-c288(w480) -> ()  [unwired: 1 out]
              }
              frame #1 {
                # "counting time"
                n305 = node-c288() -> ()  [unwired: 1 in, 1 out]
                n306 = local read "start time"() -> (w521:timestamp)
                n307 = Get Date/Time In Seconds() -> (seconds since 1Jan1904=w522:timestamp)
                n308 = property on="record channels" class="Arr (strict)"() -> ("Value"=w513:string[])  [unwired: 2 in, 2 out]
                n309 = Subtract(x=w522, y=w521) -> (x-y=w520:dbl)
                n310 = property on="connection settings" class="Clust (strict)"() -> ("Value"=w509:T10)  [unwired: 2 in, 2 out]
                n311 = for {
                  tunnel: w513 -> [w535] mode=indexing
                  tunnel: w509 -> [w531]
                  shift-right: [w534] -> w526
                  shift-left: errorcluster {"status"=FALSE, "code"=0, "source"=""} ("error out") -> [w533]
                  n312 = call "command_channel.vi"("command"=enum16{"read", "write", "reset", "conf", "link"}."reset", "channel"=w535, "error in"=w533, "connection settings"=w531) -> ("error out"=w534:errorcluster)  [unwired: 3 in, 2 out]
                }
                n313 = local read "measurement data"() -> (w525:dbl[][])
                n314 = property on="stop" class="Bool (strict)"() -> ("Value"=w516:bool)  [unwired: 2 in, 2 out]
                n315 = property on="meas time" class="DigNum (strict)"() -> ("Value"=w511:dbl)  [unwired: 2 in, 2 out]
                n316 = Not(x=w516) -> (.not. x?=w517:bool)
                n317 = Boolean To (0,1)(Boolean=w517) -> (0, 1=w515:i16)
                n318 = Multiply(x=1000.0, y=w511) -> (x*y=w512:dbl)
                n319 = Replace Array Subset(array=w525, new element=w520, index (row)=0 ("disabled index (row)"), index (col)=w524) -> (w519:dbl[][])
                n320 = Multiply(x=w512, y=w515) -> (x*y=w514:dbl)
                n321 = call <vilib>:"Clear Errors.vi"("error in (no error)"=w526) -> ()  [unwired: 5 in, 2 out]
                n322 = local write "measurement data"(w519) -> ()
                n323 = node-c288(w514) -> ()  [unwired: 1 out]
              }
              frame #2 {
                w540 = "\""
                w546 = "%#^_4G" ("format string")
                # "2D graph"
                # "3D graph"
                # "read data"
                # "measure the data"
                n324 = node-c288() -> ()  [unwired: 1 in, 2 out]
                n325 = property on="record channels" class="Arr (strict)"() -> ("Value"=w560:string[])  [unwired: 2 in, 2 out]
                n326 = property on="dimensons" class="DigNum (strict)"() -> ("Value"=w556:i32)  [unwired: 2 in, 2 out]
                n327 = Increment(x=w556) -> (x+1=w557:i32)
                n328 = for {
                  tunnel: w560 -> [w592] mode=indexing
                  tunnel: w547 -> [w589]
                  tunnel: [w585] -> w548
                  tunnel: [w579] -> w543
                  i -> [w588]
                  n329 = property on="dimensons" class="DigNum (strict)"() -> ("Value"=w586:i32)  [unwired: 2 in, 2 out]
                  n330 = property on="connection settings" class="Clust (strict)"() -> ("Value"=w583:T10)  [unwired: 2 in, 2 out]
                  n331 = Increment(x=w586) -> (x+1=w587:i32)
                  n332 = Add(x=w587, y=w588) -> (x+y=w581:i32)
                  n333 = call "command_channel.vi"("command"=enum16{"read", "write", "reset", "conf", "link"}."read", "channel"=w592, "connection settings"=w583) -> ("output"=w580:string, "error out"=w591:errorcluster)  [unwired: 4 in, 1 out]
                  n334 = Fract/Exp String To Number(use system decimal point (T)=FALSE, string=w580, default (0 dbl)=nan ("default (0 DBL)")) -> (number=w582:dbl)  [unwired: 1 in, 1 out]
                  n335 = property on="measurement data" class="Arr (strict)"() -> ("Value"=w584:dbl[][])  [unwired: 2 in, 2 out]
                  n336 = call <vilib>:"Clear Errors.vi"("error in (no error)"=w591) -> ("error out"=w579:errorcluster)  [unwired: 5 in, 1 out]
                  n337 = Replace Array Subset(array=w584, new element=w582, index (row)=w581, index (col)=w589) -> (w585:dbl[][])
                  n338 = property on="measurement data" class="Arr (strict)"("Value"=w585) -> ()  [unwired: 2 in, 2 out]
                }
                n339 = Index Array(array=w548, index (col)=w547) -> (element=w537:dbl[])  [unwired: 1 in]
                n340 = property on="set values" class="Arr (strict)"() -> ("Value"=w554:string[][])  [unwired: 2 in, 2 out]
                n341 = Array Subset(array=w537, index=1, length=w556) -> (w552:dbl[])
                n342 = Array Subset(array=w537, index=w557) -> (w558:dbl[])  [unwired: 1 in]
                n343 = for {
                  shift-right: [w572] -> w553
                  shift-left: w554 -> [w573]
                  tunnel: w546 -> [w569]
                  tunnel: w552 -> [w568] mode=indexing
                  i -> [w571]
                  n344 = Format Into String(format string=w569, w568) -> (resulting string=w567:string)  [unwired: 2 in, 1 out]
                  n345 = Replace Array Subset(array=w573, new element=w567, index (row)=w571, index (col)=1 ("disabled index (col)")) -> (w572:string[][])
                }
                n346 = for {
                  tunnel: w558 -> [w576] mode=indexing
                  tunnel: [w575] -> w551 mode=indexing
                  tunnel: w546 -> [w574]
                  n347 = Format Into String(format string=w574, w576) -> (resulting string=w575:string)  [unwired: 2 in, 1 out]
                }
                n348 = for {
                  tunnel: w537 -> [w562] mode=indexing
                  tunnel: w546 -> [w563]
                  tunnel: [w561] -> w536 mode=indexing
                  n349 = Format Into String(format string=w563, w562) -> (resulting string=w561:string)  [unwired: 2 in, 1 out]
                }
                n350 = property on="set values" class="Arr (strict)"("Value"=w553) -> ()  [unwired: 2 in, 2 out]
                n351 = property on="auto update" class="Bool (strict)"() -> ("Value"=w550:bool)  [unwired: 2 in, 2 out]
                n352 = property on="column separator" class="Str"() -> ("Value"=w545:string)  [unwired: 2 in, 2 out]
                n353 = Array To Spreadsheet String(delimiter (Tab)=w545, array=w536, 3:"%s" ("format string")) -> (spreadsheet string=w539:string)
                "data" <- w539
                n354 = case shown="True" w550 {
                  frame False {
                  }
                  frame True {
                    n355 = property on="3D graph parameters" class="Clust (strict)"() -> ("Value"=w564:T11)  [unwired: 2 in, 2 out]
                    n356 = property on="3D graph parameters" class="Clust (strict)"("Val(Sgnl)"=w564) -> ()  [unwired: 2 in, 2 out]
                  }
                }
                n357 = Concatenate Strings(w540, w539, w540) -> (w538:string)
                n358 = property on="auto update" class="Bool (strict)"() -> ("Value"=w549:bool)  [unwired: 2 in, 2 out]
                n359 = call "command_channel.vi"("command"=T15."write", "channel"="data", "data"=w538, "error in"=w543) -> ()  [unwired: 3 in, 3 out]
                n360 = case shown="True" w549 {
                  tunnel: w551 -> [w565 w566]
                  frame False {
                    n361 = property on="latest" class="Arr (strict)"("Value"=w565) -> ()  [unwired: 2 in, 2 out]
                  }
                  frame True {
                    n362 = property on="latest" class="Arr (strict)"("Val(Sgnl)"=w566) -> ()  [unwired: 2 in, 2 out]
                  }
                }
                n363 = node-c288() -> ()  [unwired: 1 in, 1 out]
              }
            }
          }
          n364 = node-c288(w447) -> ()  [unwired: 2 out]
          n365 = property on="save measurement" class="Bool (strict)"() -> ("Value"=w449:bool)  [unwired: 2 in, 2 out]
          n366 = call "command_channel.vi"() -> ()  [unwired: 7 in, 3 out]
        }
        n367 = Transpose 2D Array(2D array=w302) -> (transposed array=w285:dbl[][])
        n368 = flat-sequence {
          tunnel: w274 -> [_]
          tunnel: [w349] -> w275
          tunnel: w275 -> [w353]
          frame #0 {
            n369 = property on="dimensons" class="DigNum (strict)"() -> ("Value"=w339:i32)  [unwired: 2 in, 2 out]
            n370 = for {
              N: w339 -> [_]
              i -> [w342]
              n371 = property on="scan" class="Arr (strict)"() -> ("Value"=w343:T5)  [unwired: 2 in, 2 out]
              n372 = Index Array(array=w343, index=w342) -> (element=w341:T19)
              n373 = Unbundle By Name(w341) -> ("set channel"=w346:string)
              n374 = call "command_channel.vi"("command"=enum16{"read", "write", "reset", "conf", "link"}."write", "channel"=w346, "data"="0") -> ("error out"=w345:errorcluster)  [unwired: 4 in, 2 out]
              n375 = call <vilib>:"Clear Errors.vi"("error in (no error)"=w345) -> ()  [unwired: 5 in, 2 out]
            }
          }
          frame #1 {
            n376 = property on="measurement end commands" class="Str"() -> ("Value"=w348:string)  [unwired: 2 in, 2 out]
            n377 = property on="connection settings" class="Clust (strict)"() -> ("Value"=w347:T10)  [unwired: 2 in, 2 out]
            n378 = Concatenate Strings(w348, "\r\n") -> (w350:string)
            n379 = call "command_channel.vi"("command"=T15."raw communication", "data"=w350, "connection settings"=w347) -> ("error out"=w349:errorcluster)  [unwired: 4 in, 2 out]
          }
          frame #2 {
            n380 = call <vilib>:"Clear Errors.vi"("error in (no error)"=w353) -> ()  [unwired: 5 in, 2 out]
            n381 = property on="Y channels" class="Arr (strict)"() -> ("Value"=w355:u16[])  [unwired: 2 in, 2 out]
            n382 = for {
              tunnel: w355 -> [w368] mode=indexing
              tunnel: [w365] -> w356 mode=indexing
              n383 = local read "measurement data"() -> (w369:dbl[][])
              n384 = property on="X channel" class="Ring (strict)"() -> ("Value"=w364:u16)  [unwired: 2 in, 2 out]
              n385 = Index Array(array=w369, index (row)=w364) -> (element=w366:dbl[])  [unwired: 1 in]
              n386 = Index Array(array=w369, index (row)=w368) -> (element=w367:dbl[])  [unwired: 1 in]
              n387 = Bundle("measurement data"=w366, "measurement data"=w367) -> (w365:T14)  [unwired: 1 in]
            }
            n388 = local read "graph history"() -> (w359:T1)
            n389 = property on="graph history" class="DigNum (strict)"() -> ("Value"=w354:i32)  [unwired: 2 in, 2 out]
            n390 = Build Array (concatenate)(w359, w356) -> (w358:T1)
            n391 = Array Size(array=w356) -> (size(s)=w362:i32)
            n392 = Array Size(array=w358) -> (size(s)=w363:i32)
            n393 = Multiply(x=w362, y=w354) -> (x*y=w361:i32)
            n394 = Subtract(x=w363, y=w361) -> (x-y=w357:i32)
            n395 = Array Subset(array=w358, index=w357, length=w361) -> (→"graph history":T1)
          }
          frame #3 {
            n396 = property on="load next" class="Bool (strict)"() -> ("Value"=w370:bool)  [unwired: 2 in, 2 out]
            n397 = case shown="True" w370 {
              frame False {
              }
              frame True {
                # "LOAD default configuration on startup"
                n398 = property on="next configuration" class="CmbBox"() -> ("Value"=w371:string)  [unwired: 2 in, 2 out]
                n399 = property on="program path" class="Path"() -> ("Value"=w375:path)  [unwired: 2 in, 2 out]
                n400 = property on="Configuration" class="CmbBox"("Value"=w371) -> ()  [unwired: 2 in, 2 out]
                n401 = Concatenate Strings(w371, ".pnl" ("string")) -> (w374:string)
                n402 = Build Path(base path=w375, name or relative path=w374) -> (appended path=w372:path)
                n403 = property on="saved controls" class="Arr (strict)"() -> ("Value"=w376:string[])  [unwired: 2 in, 2 out]
                n404 = control-ref of="This VI"() -> (w377:refnum<vi>)
                n405 = call "front_panel_ctl_save.vi"("VI in"=w377, "method"=enum16{"read controls", "write controls"}."read controls", "filename"=w372, "controls"=w376) -> ("error out"=w379:errorcluster)  [unwired: 4 in]
                n406 = call <vilib>:"Clear Errors.vi"("error in (no error)"=w379) -> ()  [unwired: 5 in, 2 out]
              }
            }
          }
        }
        n407 = case shown="True" w274 {
          tunnel: w285 -> [_ w388]
          tunnel: w260 -> [_ w385]
          frame False {
          }
          frame True {
            n408 = flat-sequence {
              tunnel: w398 -> [w410]
              tunnel: [w406] -> w391
              frame #0 {
                n409 = Get Date/Time In Seconds() -> (seconds since 1Jan1904=w411:timestamp)
                n410 = Unbundle By Name(w410) -> ("measurement file"=w412:string)
                n411 = property on="program path" class="Path"() -> ("Value"=w405:path)  [unwired: 2 in, 2 out]
                n412 = Format Date/Time String(time format string (%c)=w412, seconds (now)=w411) -> (date/time string=w413:string)  [unwired: 1 in]
                n413 = Build Path(base path=w405, name or relative path=w413) -> (appended path=w407:path)
                n414 = Strip Path(path=w407) -> (stripped path=w409:path)  [unwired: 1 out]
                n415 = Path To String(path=w407) -> (string=w406:string)
                n416 = Create Folder(path (use dialog)=w409) -> (error out=w408:errorcluster)  [unwired: 2 in, 2 out]
                n417 = call <vilib>:"Clear Errors.vi"("error in (no error)"=w408) -> ()  [unwired: 5 in, 2 out]
              }
            }
            n418 = local read "measurement logging"() -> (w398:T8)
            n419 = Concatenate Strings(w391, ".csv" ("name or relative path")) -> (w394:string)
            n420 = String To Path(string=w394) -> (path=w395:path)
            n421 = Open/Create/Replace File(file path (use dialog)=w395, operation (0:open)=T12."open or create") -> (refnum out=w401:refnum<file>, error out=w403:errorcluster)  [unwired: 4 in, 1 out]
            n422 = Set File Position(refnum=w401, from (0:start)=enum16{"start", "end", "current"}."end", error in=w403) -> (refnum out=w399:refnum<file>, error out=w400:errorcluster)  [unwired: 1 in]
            n423 = Concatenate Strings(w391, ".log" ("name or relative path")) -> (w390:string)
            n424 = property on="logged controls" class="Arr (strict)"() -> ("Value"=w387:refnum<vi>[])  [unwired: 2 in, 2 out]
            n425 = String To Path(string=w390) -> (path=w389:path)
            n426 = call "log_controls.vi"("Controls[]"=w387, "filename"=w389) -> ()  [unwired: 6 in, 1 out]
            n427 = Increment(x=w385) -> (x+1=w386:i32)
            n428 = for {
              N: w386 -> [_]
              tunnel: w388 -> [w418] mode=indexing
              shift-right: [w431] -> w396
              shift-left: w399 -> [w424]
              shift-right: [w430] -> w397
              shift-left: w400 -> [w423]
              n429 = property on="column separator" class="Str"() -> ("Value"=w415:string)  [unwired: 2 in, 2 out]
              n430 = local read "start time"() -> (w429:timestamp)
              n431 = Index Array(array=w418, index=0) -> (element=w419:dbl)
              n432 = Concatenate Strings("%Y-%m-%dT%H:%M:%S" ("time format string (%c)"), w415) -> (w416:string)
              n433 = Add(x=w429, y=w419) -> (x+y=w428:timestamp)
              n434 = Format Date/Time String(time format string (%c)=w416, seconds (now)=w428) -> (date/time string=w421:string)  [unwired: 1 in]
              n435 = Write to Text File(file (use dialog)=w424, text=w421, error in=w423) -> (refnum out=w426:refnum<file>, error out=w425:errorcluster)  [unwired: 1 in, 1 out]
              n436 = for {
                tunnel: w418 -> [w437] mode=indexing
                shift-right: [w440] -> w432
                shift-left: w426 -> [w438]
                shift-right: [w441] -> w427
                shift-left: w425 -> [w439]
                tunnel: w415 -> [w436]
                tunnel: "%#^_4G" ("format string") -> [w435]
                n437 = Concatenate Strings(w435, w436) -> (w434:string)
                n438 = Format Into String(format string=w434, w437) -> (resulting string=w433:string)  [unwired: 2 in, 1 out]
                n439 = Write to Text File(file (use dialog)=w438, text=w433, error in=w439) -> (refnum out=w440:refnum<file>, error out=w441:errorcluster)  [unwired: 1 in, 1 out]
              }
              n440 = Write to Text File(file (use dialog)=w432, text="\r\n", error in=w427) -> (refnum out=w431:refnum<file>, error out=w430:errorcluster)  [unwired: 1 in, 1 out]
            }
            n441 = Close File(refnum=w396, error in=w397) -> ()  [unwired: 2 out]
          }
        }
      }
    }
    n442 = local write "stop"(w255) -> ()
  }
